vi "Formating 2D Barcode 2.0.vi"(8 "Plant Number":u8 max=9, 10 "Serial Number":string, 11 "IRS Number":string) -> (2 "2-D Barcode":string)   [LabVIEW 2018]
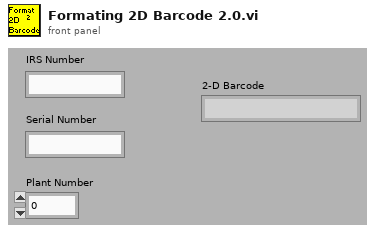
[diagram p1: front panel]
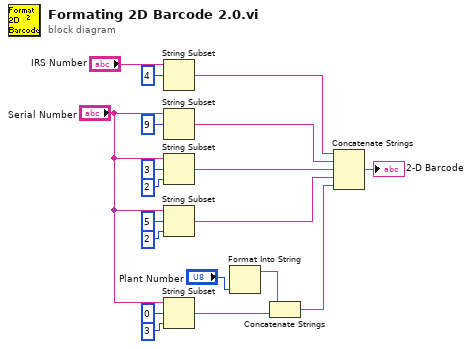
[diagram p0: block diagram]
diagram:
  n1 = String Subset(string="IRS Number", offset (0)=4) -> (substring=w8:string)  [unwired: 1 in]
  n2 = String Subset(string="Serial Number", offset (0)=9) -> (substring=w7:string)  [unwired: 1 in]
  n3 = String Subset(string="Serial Number", offset (0)=3, length (rest)=2 ("length (rest)")) -> (substring=w6:string)
  n4 = String Subset(string="Serial Number", offset (0)=5, length (rest)=2 ("length (rest)")) -> (substring=w5:string)
  n5 = String Subset(string="Serial Number", offset (0)=0, length (rest)=3 ("length (rest)")) -> (substring=w15:string)
  n6 = Format Into String("Plant Number") -> (resulting string=w1:string)  [unwired: 3 in, 1 out]
  n7 = Concatenate Strings(w1, w15) -> (w4:string)
  n8 = Concatenate Strings(w8, w7, w6, w5, w4) -> (→"2-D Barcode":string)
